vi "Program21.vi"() -> ()   [LabVIEW 2020]
panel:
  out "Array":dbl[](array[numeric])
  out "Wynik fun Replace":dbl[](array[numeric])
  out "initialized array":dbl[](array[numeric])
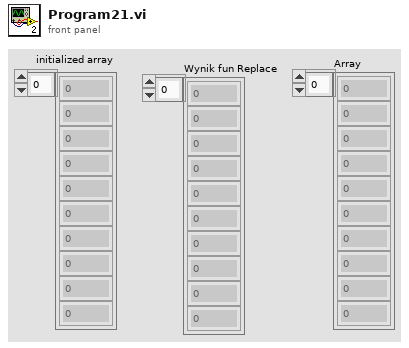
[diagram p1: front panel]
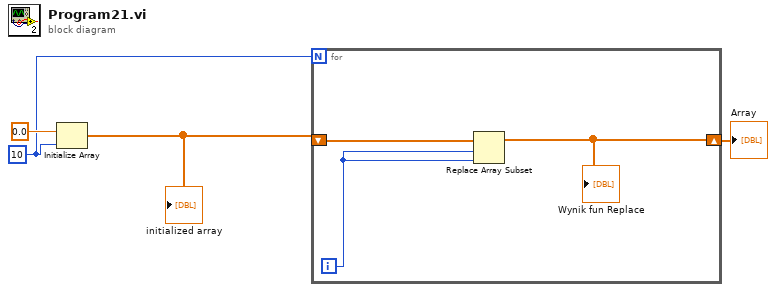
[diagram p0: block diagram]
diagram:
  w3 = 10 ("dimension size")
  n1 = Initialize Array(0.0 ("element"), w3) -> (w2:dbl[])
  "initialized array" <- w2
  n2 = for {
    N: w3 -> [_]
    shift-right: [w5] -> w1
    shift-left: w2 -> [w7]
    i -> [w6]
    n3 = Replace Array Subset(array=w7, new element=w6, index=w6) -> (w5:dbl[])
    "Wynik fun Replace" <- w5
  }
  "Array" <- w1
